vi "Entry.vi"(8 "error in (no error)":errorcluster, 11 "New State":refnum<class "Command Processor.lvclass">) -> (0 "error out":errorcluster, 3 "State out":refnum<class "Command Processor.lvclass">)   [LabVIEW 2013, in "Command Processor.lvlib" / "Command Processor.lvclass"]
doc: "This is an abstract method. Override this method to define the behavior when you enter the state."
uses:
  Command Processor.lvclass
  <vilib>/ni/Actors/State Actor/State Actor/State Actor.lvclass
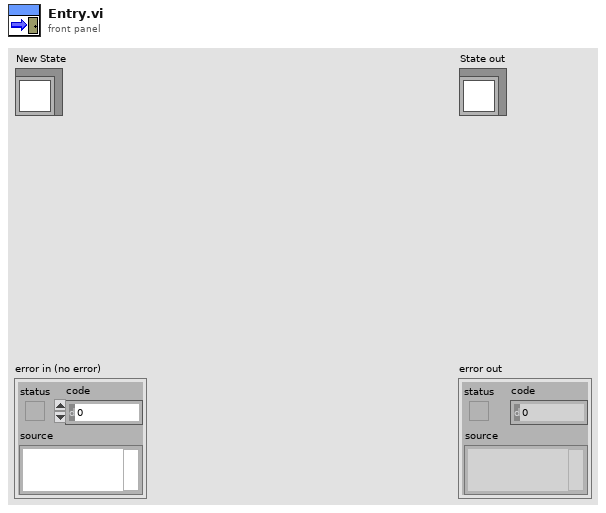
[diagram p1: front panel]
types:
  T1 = typedef "Command Processor.lvlib/Command Processor.lvclass/Command Processor Status.ctl" = cluster{"State Entry time":timestamp, "State Status":T2, "Command Processor Current State":string, "Command Status":T4}
  T2 = typedef "Current Previous State Status.ctl" = cluster{"Current State Status":T3, "Previous State Status":T3}
  T3 = typedef "State Status.ctl" = cluster{"State Name":string, "State Entry Time":timestamp, "State Exit Time":timestamp}
  T4 = typedef "Command Processor.lvlib/Command.lvlib/Command.lvclass/Command Status.ctl" = cluster{"Command Name":string, "Current State Status":T5, "Command Start Time":timestamp, "Command End Time":timestamp, "Previous State Status":T5}
  T5 = typedef "Command Processor.lvlib/Command.lvlib/Command.lvclass/State Status.ctl" = cluster{"State Name":string, "State Entry Time":timestamp, "State Exit Time":timestamp}
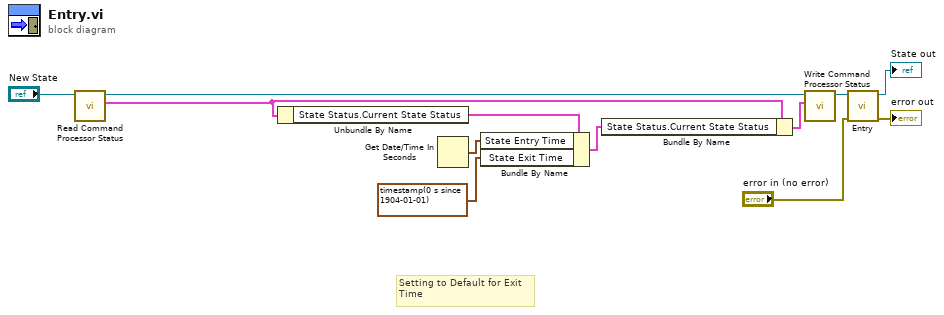
[diagram p0: block diagram]
diagram:
  # "Setting to Default for Exit \nTime"
  n1 = call-dynamic "Read Command Processor Status.vi"("Command Processor in"="New State") -> ("Command Processor Status"=w5:T1, "Command Processor out"=w9:refnum<class "Command Processor.lvclass">)  [unwired: 8 in, 1 out]
  n2 = Unbundle By Name(w5) -> ("State Status.Current State Status"=w4:T3)
  n3 = Get Date/Time In Seconds() -> (seconds since 1Jan1904=w2:timestamp)
  n4 = Bundle By Name(cluster=w4, "State Entry Time"=w2, "State Exit Time"=timestamp(0 s since 1904-01-01)) -> (w3:T3)
  n5 = Bundle By Name(cluster=w5, "State Status.Current State Status"=w3) -> (w7:T1)
  n6 = call-dynamic "Write Command Processor Status.vi"("Command Processor Status"=w7, "Command Processor in"=w9) -> ("Command Processor out"=w8:refnum<class "Command Processor.lvclass">)  [unwired: 8 in, 1 out]
  n7 = call-parent "Entry.vi"("error in (no error)"="error in (no error)", "New State"=w8) -> ("error out"=→"error out":errorcluster, "State out"=→"State out":refnum<class "Command Processor.lvclass">)  [unwired: 8 in]
